vi "StarttoGoalLine.vi"(11 "startgoal_calcout":cluster{"x0":i32, "x1":i32, "y1":i32, "y0":i32}) -> (0 "y Line coords":i32[](array[numeric]), 1 "x Line coords":i32[](array[numeric]))   [LabVIEW 2013]
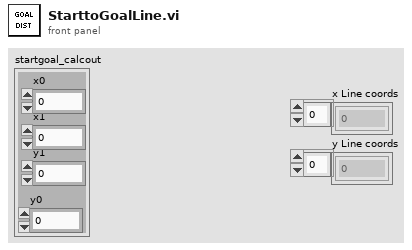
[diagram p1: front panel]
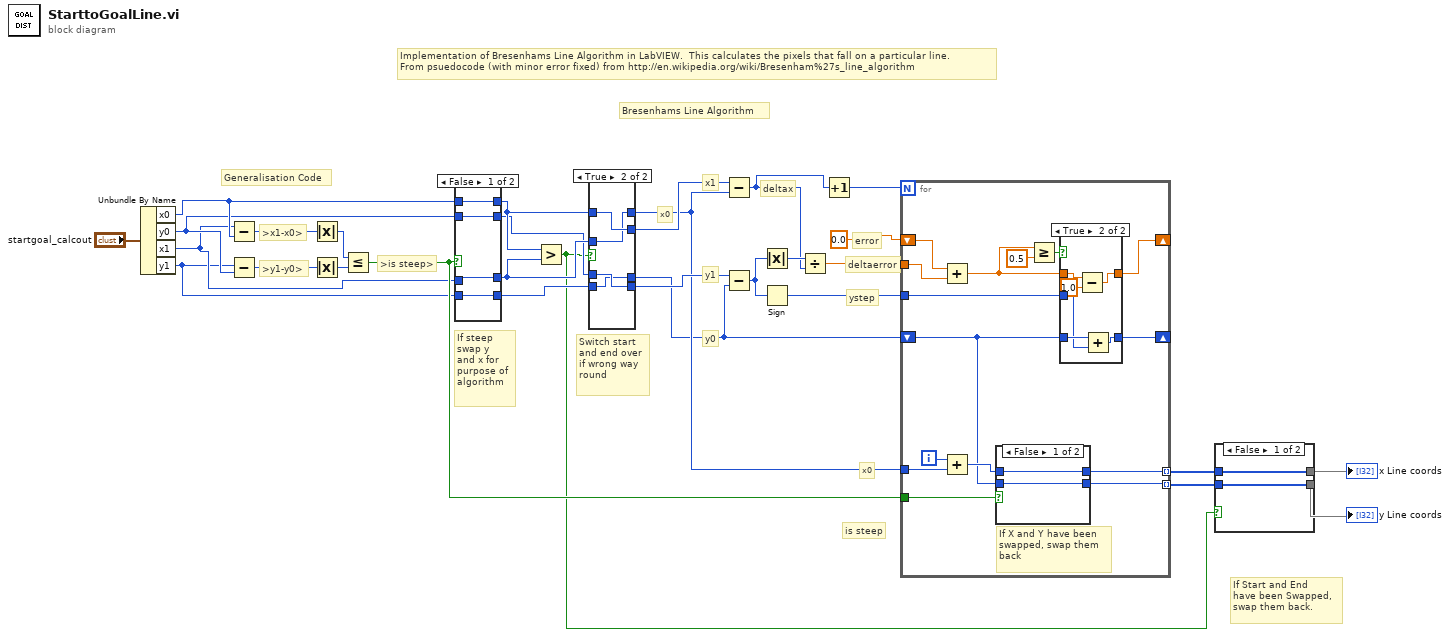
[diagram p0: block diagram]
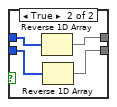
[diagram p2: hidden frame]
diagram:
  # "Bresenhams Line Algorithm"
  # "If Start and End\nhave been Swapped,\nswap them back."
  # "Implementation of Bresenhams Line Algorithm in LabVIEW.  This calculates the pixels that fall on a particular line.\nFrom psuedocode (with minor error fixed) from http://en.wikipedia.org/wiki/Bresenham%27s_line_algorithm"
  # "Switch start\nand end over\nif wrong way\nround"
  # "If steep\nswap y\nand x for\npurpose of\nalgorithm"
  # "is steep"
  # "x0"
  # "Generalisation Code"
  # "y0"
  # "deltaerror"
  # "error"
  # "ystep"
  # "deltax"
  # "y1"
  # "x1"
  # "x0"
  # ">is steep>"
  # ">y1-y0>"
  # ">x1-x0>"
  n1 = Unbundle By Name("startgoal_calcout") -> ("x0"=w4:i32, "y0"=w3:i32, "x1"=w2:i32, "y1"=w1:i32)
  n2 = Subtract(x=w2, y=w4) -> (x-y=w30:i32)
  n3 = Subtract(x=w1, y=w3) -> (x-y=w29:i32)
  n4 = Absolute Value(x=w30) -> (abs(x)=w27:i32)
  n5 = Absolute Value(x=w29) -> (abs(x)=w28:i32)
  n6 = Less Or Equal?(x=w27, y=w28) -> (x <= y?=w13:bool)
  n7 = case shown="False" w13 {
    tunnel: w4 -> [w34 w38]
    tunnel: w2 -> [w33 w37]
    tunnel: w3 -> [w32 w36]
    tunnel: w1 -> [w31 w35]
    tunnel: [w32 w38] -> w24
    tunnel: [w31 w37] -> w23
    tunnel: [w34 w36] -> w26
    tunnel: [w33 w35] -> w25
    frame False {
    }
    frame True {
    }
  }
  n8 = Greater?(x=w26, y=w25) -> (0:w10:bool)
  n9 = case shown="True" w10 {
    tunnel: w26 -> [w42 w46]
    tunnel: w25 -> [w41 w45]
    tunnel: w24 -> [w40 w44]
    tunnel: w23 -> [w39 w43]
    tunnel: [w42 w45] -> w18
    tunnel: [w41 w46] -> w22
    tunnel: [w40 w43] -> w15
    tunnel: [w39 w44] -> w21
    frame False {
    }
    frame True {
    }
  }
  n10 = Subtract(x=w22, y=w18) -> (x-y=w12:i32)
  n11 = Subtract(x=w21, y=w15) -> (x-y=w19:i32)
  n12 = Absolute Value(x=w19) -> (abs(x)=w20:i32)
  n13 = Sign(1:w19) -> (0:w14:i32)
  n14 = Divide(x=w20, y=w12) -> (x/y=w16:dbl)
  n15 = Increment(x=w12) -> (x+1=w11:i32)
  n16 = for {
    N: w11 -> [_]
    tunnel: w18 -> [w60]
    shift-right: [w50] -> _
    shift-left: 0.0 -> [w51]
    tunnel: w16 -> [w59]
    tunnel: w14 -> [w53]
    tunnel: w13 -> [w58]
    shift-right: [w52] -> _
    shift-left: w15 -> [w54]
    tunnel: [w48] -> w9 mode=indexing
    tunnel: [w47] -> w8 mode=indexing
    i -> [w61]
    # "If X and Y have been\nswapped, swap them\nback"
    n17 = Add(x=w51, y=w59) -> (x+y=w49:dbl)
    n18 = Add(x=w61, y=w60) -> (x+y=w57:i32)
    n19 = case shown="False" w58 {
      tunnel: w54 -> [w70 w73]
      tunnel: [w71 w73] -> w48
      tunnel: w57 -> [w71 w72]
      tunnel: [w70 w72] -> w47
      frame False {
      }
      frame True {
      }
    }
    n20 = Greater Or Equal?(x=w49, y=0.5) -> (x >= y?=w56:bool)
    n21 = case shown="True" w56 {
      tunnel: w54 -> [w62 w69]
      tunnel: w53 -> [_ w66]
      tunnel: [w62 w68] -> w52
      tunnel: w49 -> [w63 w67]
      tunnel: [w63 w65] -> w50
      frame False {
      }
      frame True {
        n22 = Subtract(x=w67, y=1.0) -> (x-y=w65:dbl)
        n23 = Add(x=w69, y=w66) -> (x+y=w68:i32)
      }
    }
  }
  n24 = case shown="False" w10 {
    tunnel: [w75 w79] -> w7
    tunnel: w9 -> [w75 w78]
    tunnel: w8 -> [w74 w77]
    tunnel: [w74 w76] -> w6
    frame False {
    }
    frame True {
      n25 = Reverse 1D Array(array=w78) -> (reversed array=w79:i32[])
      n26 = Reverse 1D Array(array=w77) -> (reversed array=w76:i32[])
    }
  }
  "x Line coords" <- w7
  "y Line coords" <- w6
